vi "LVFunction_Imop_WavefrontCorrectorStateFile_GetInformation.vi"(0 "path":path, 11 "error in (no error)":errorcluster) -> (4 "path (dup)":path, 6 "Actuators":i32, 15 "error out":errorcluster)   [LabVIEW 2018]
doc: "Wavefront corrector parameter getter for parameter of type boolean.\n\n--------------------------------------------------------------------------------\n\n<B>correctorIn </B> : WavefrontCorrector object.\n<B>correctorOut </B> : WavefrontCorrector object.\n<B>parameter_name </B> : Name of the parameter.\n<B>value </B> : Value of the parameter.\n<B>ErrorIn </B> : Error\n<B>ErrorOut </B> : Error\n\n--------------------------------------------------------------------------------"
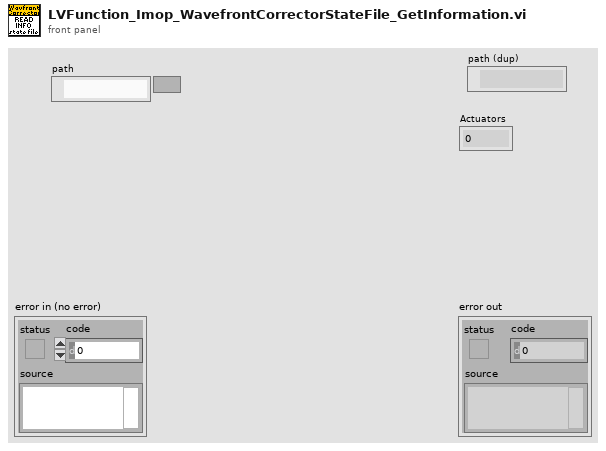
[diagram p1: front panel]
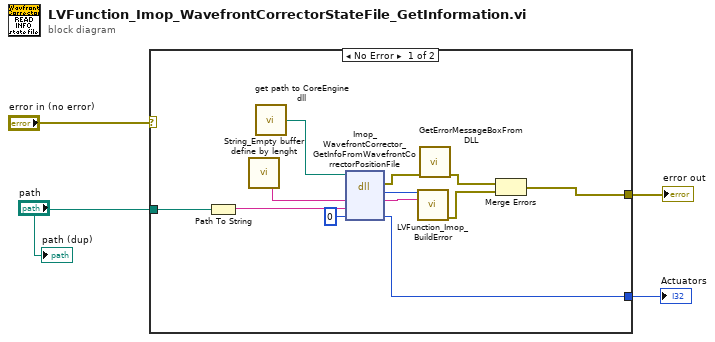
[diagram p0: block diagram]
diagram:
  n1 = case shown="No Error" "error in (no error)" {
    selector: "error in (no error)" -> [_ w17]
    tunnel: [w9 w17] -> w3
    tunnel: "path" -> [w7 _]
    tunnel: [w6 _] -> w2
    frame No Error {
      n2 = Path To String(path=w7) -> (string=w8:string)
      n3 = call "String_Empty buffer define by lenght.vi"() -> ("Empty buffer"=w12:string)  [unwired: 1 in]
      n4 = call "get path to CoreEngine dll.vi"() -> ("path to wavekit library"=w14:path)  [unwired: 14 in, 1 out]
      n5 = dll-call lib="D:/SOFTware/CoreEngine4_Suite/SVN_trunk/LV2011_interface/DLLs/c_interface_vc100.dll" fn="Imop_WavefrontCorrector_GetInfoFromWavefrontCorrectorPositionFile"(path in=w14, "message"=w12, "file_path"=w8, "nb_actuators"=0) -> (error out=w13:errorcluster, "return type"=w16:i32, "message"=w15:string, "nb_actuators"=w6:i32)  [unwired: 3 in, 1 out]
      n6 = call "LVFunction_Imop_BuildError.vi"("code"=w16, "String to Prepend to source (\"\")"=w15) -> ("error out"=w10:errorcluster)  [unwired: 13 in]
      n7 = call "GetErrorMessageBoxFromDLL.vi"("error IN"=w13) -> ("error OUT"=w11:errorcluster)  [unwired: 10 in]
      n8 = Merge Errors(w11, w10) -> (w9:errorcluster)
    }
    frame Error {
    }
  }
  "error out" <- w3
  "Actuators" <- w2
  "path (dup)" <- "path"
